vi "Write Maximum Frequency.vi"(10 "Maximum Frequency":dbl, 11 "Spectrum Analyzer in":refnum<class "Spectrum Analyzer.lvclass">) -> (3 "Spectrum Analyzer out":refnum<class "Spectrum Analyzer.lvclass">)   [LabVIEW 2020, in "Spectrum Analyzer.lvclass"]
uses:
  Spectrum Analyzer.lvclass
  Spectrum Analyzer.lvclass/Spectrum Analyzer.ctl
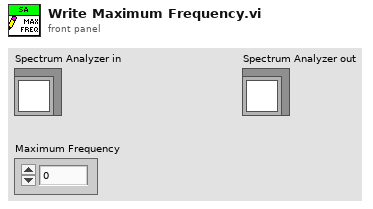
[diagram p1: front panel]
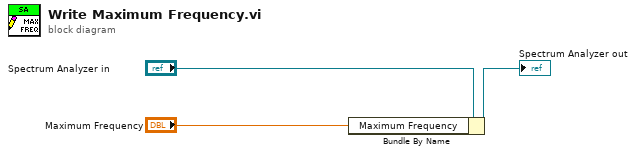
[diagram p0: block diagram]
diagram:
  n1 = Bundle By Name(cluster="Spectrum Analyzer in", "Maximum Frequency"="Maximum Frequency") -> (→"Spectrum Analyzer out":refnum<class "Spectrum Analyzer.lvclass">)
